vi "Aim Rotation.vi"() -> (2 "Rotation":dbl, 3 "Image Size X":dbl)   [LabVIEW 2016]
uses:
  <vilib>/Rock Robotics/Network Tables/NT Read Number.vi
  <vilib>/Rock Robotics/Network Tables/NT Read Boolean.vi
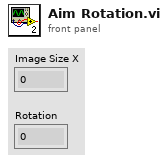
[diagram p1: front panel]
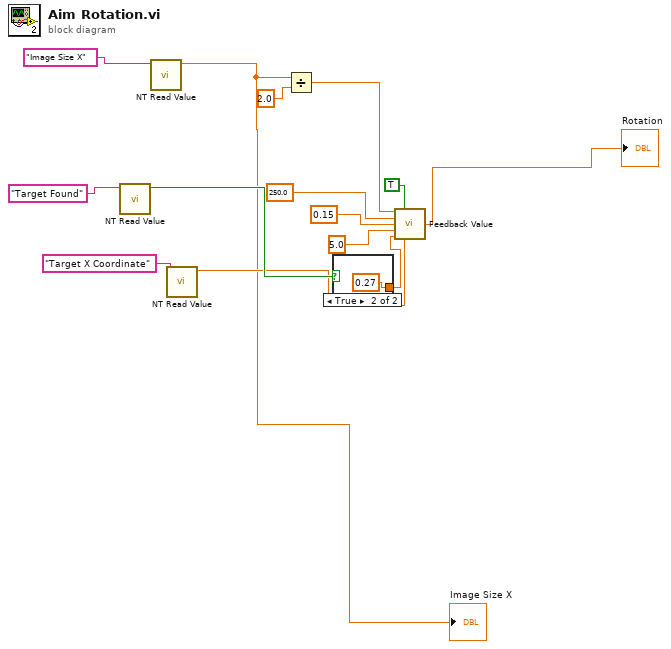
[diagram p0: block diagram]
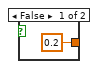
[diagram p2: hidden frame]
diagram:
  n1 = call-poly <vilib>:"NT Read Value.vi"("Name"="Target Found") -> ("Boolean"=w13:bool)  [unwired: 9 in, 1 out]
  n2 = call-poly <vilib>:"NT Read Value.vi"("Name"="Image Size X") -> ("Numeric"=w9:dbl)  [unwired: 9 in, 1 out]
  "Image Size X" <- w9
  n3 = call-poly <vilib>:"NT Read Value.vi"("Name"="Target X Coordinate") -> ("Numeric"=w11:dbl)  [unwired: 9 in, 1 out]
  n4 = Divide(x=w9, y=2.0) -> (x/y=w6:dbl)
  n5 = case shown="True" w13 {
    tunnel: [0.2 ("Maximum Amplitude") 0.27 ("Maximum Amplitude")] -> w2
    frame False {
    }
    frame True {
    }
  }
  n6 = call "Feedback Value.vi"("Set Point"=w6, "Invert Rotation"=TRUE, "Divisor"=250.0, "Addend"=0.15, "Deadband"=5.0, "Maximum Amplitude"=w2, "Current Value"=w11) -> ("Rotation"=→"Rotation":dbl)  [unwired: 8 in]
